vi "Actor Core.vi"(8 "error in":errorcluster, 11 "Launch IMAQ Display in":refnum<class "Launch IMAQ Display.lvclass">) -> (0 "error out":errorcluster, 3 "Actor out":refnum<class "Actor.lvclass">)   [LabVIEW 2014, in "Launch IMAQ Display.lvlib" / "Launch IMAQ Display.lvclass"]
doc: "(<B>Filename</B>: Actor Framework.lvlib:Actor.lvclass:Actor Core.vi)\n\nReceives messages to the actor, reacts to them, and initiates any error handling that may shut the actor down.\n\nDescendant classes may override this VI to append parallel tasks for the actor to complete while it handles messages. Overrides use the Call Parent Method node."
uses:
  Launch IMAQ Display.lvclass
  <vilib>/ActorFramework/Actor/Actor.lvclass
  HIJ IMAQdx Display/AF IMAQ Display/HIJ IMAQdx Display.lvclass
  Analyze Classes/Analyze Diviation/Analyze BeamDeviation.lvclass
  Results and Overlays/Results Beam Deviation/Analyze Results Beam Deviation.lvclass
  Analyze Classes/Analyze Distanz/Analyze Distanz.lvclass
  Results and Overlays/Results Distance/Analyze Results Distanz.lvclass
  IMAQdx Actor/IMAQdx Actor/IMAQdx Actor.lvclass
  Analyze Classes/Analyze Fluence/Analyze Fluence.lvclass
  Results and Overlays/Results Fluence/Analyze Results Fluence.lvclass
  Results and Overlays/Results Base/Analyze Results Base.lvclass/Analyze Results Base.ctl
  Results and Overlays/Results Fluence/Analyze Results Fluence.lvclass/Analyze Results Fluence.ctl
  HIJ Vision Display/HIJ Vision Display/HIJ Vision Display.lvclass/HIJ Vision Display.ctl
  Applications/HIJ Vision Application/HIJ Vision Application/HIJ Vision Application.lvclass/HIJ Vision Application.ctl
  Applications/HIJ Vision Camera App/HIJ Vision Camera App/HIJ Vision Camera App.lvclass/HIJ Vision Camera App.ctl
  <vilib>/ActorFramework/Actor/Actor.lvclass/Actor.ctl
  <vilib>/ActorFramework/Message Enqueuer/Message Enqueuer.lvclass/Message Enqueuer.ctl
  Applications/HIJ Vision Camera App/HIJ Vision Camera App Messages/Menu Selection Msg/Menu Selection Msg.lvclass/Menu Selection Msg.ctl
  Results and Overlays/Results Base/Write Overlay_.vi
  Results and Overlays/Results Base/Write Overlay colors.vi
  Results and Overlays/Results Fluence/Write UI Ref Max F.vi
  HIJ Vision Display/HIJ Vision Display/Write Save Report_.vi
  Applications/HIJ Vision Application/HIJ Vision Application/Write SubPnl for Display.vi
  Applications/HIJ Vision Camera App/HIJ Vision Camera App/Write Child Menu.vi
  Applications/HIJ Vision Application/HIJ Vision Application/Write HIJ Vision Display.vi
  Applications/HIJ Vision Application/HIJ Vision Application/Write Analyze Objs.vi
  Applications/HIJ Vision Camera App/HIJ Vision Camera App/Write Camera Actor.vi
  Applications/HIJ Vision Camera App/HIJ Vision Camera App/Write SubPnl for Settings.vi
  <vilib>/ActorFramework/Message Enqueuer/Init from Existing Queue.vi
  <vilib>/ActorFramework/Message Enqueuer/Enqueue.vi
  <vilib>/ActorFramework/Message Priority Queue/Priority Enqueue.vi
  <vilib>/ActorFramework/Message Enqueuer/Message Enqueuer.lvclass
  Applications/HIJ Vision Camera App/HIJ Vision Camera App Messages/Menu Selection Msg/Menu Selection Msg.lvclass
  <vilib>/ActorFramework/Stop Msg/Stop Msg.lvclass
  Applications/HIJ Vision Camera App/HIJ Vision Camera App/HIJ Vision Camera App.lvclass
panel:
  out "Max Fluence":dbl[unit]
  in  "Stop Button":bool
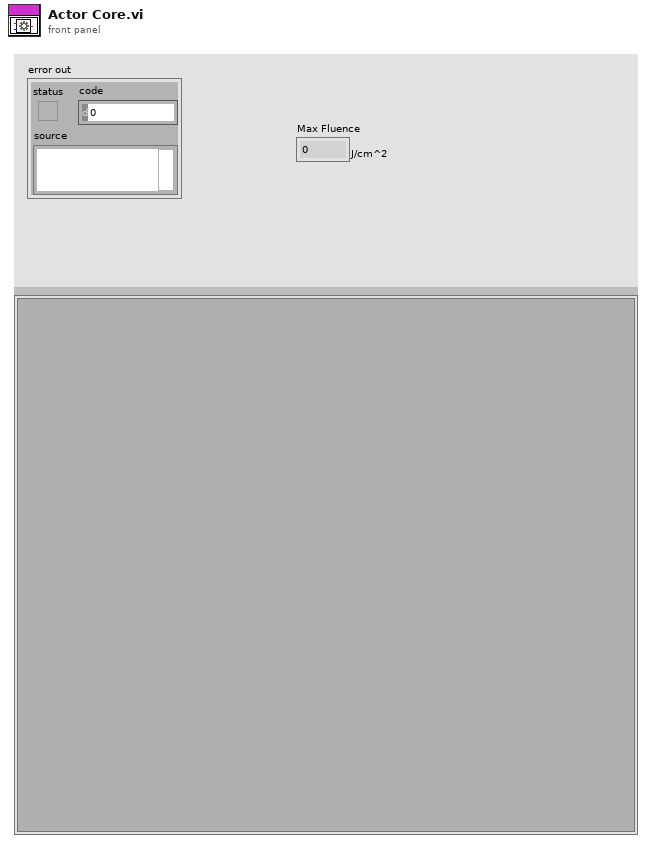
[diagram p1: front panel]
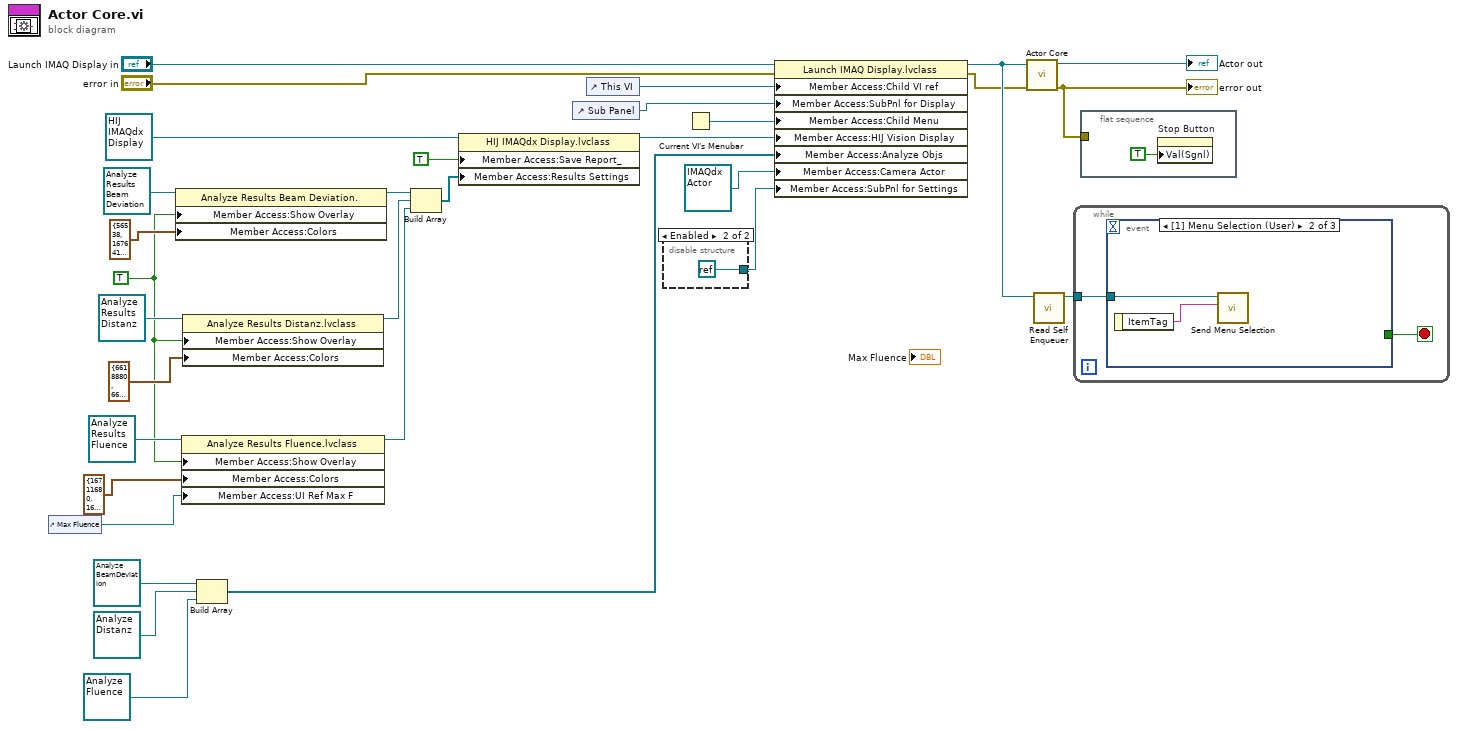
[diagram p0: block diagram]
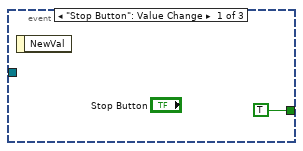
[diagram p3: hidden frame]
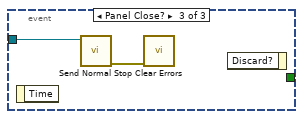
[diagram p4: hidden frame]
diagram:
  w3 = TRUE ("bOverlay")
  n1 = control-ref of="Max Fluence"() -> (w1:refnum<vi>)
  n2 = property class="Analyze Results Beam Deviation."(reference=refnum<class "Analyze Results Beam Deviation.lvclass"> refnum ("Analyze Results Beam Deviation.lvclass"), "Member Access:Show Overlay"=w3, "Member Access:Colors"=cluster{"Border":u32, "Text":u32} {"Border"=56538, "Text"=16764160} ("Colors")) -> (reference out=w23:refnum<class "Analyze Results Beam Deviation.lvclass">)  [unwired: 1 in, 1 out]
  n3 = property class="Analyze Results Fluence.lvclass"(reference=refnum<class "Analyze Results Fluence.lvclass"> refnum ("Analyze Results Fluence.lvclass"), "Member Access:Show Overlay"=w3, "Member Access:Colors"=cluster{"Border":u32, "Text":u32} {"Border"=16711680, "Text"=16448250} ("Colors"), "Member Access:UI Ref Max F"=w1) -> (reference out=w4:refnum<class "Analyze Results Fluence.lvclass">)  [unwired: 1 in, 1 out]
  n4 = property class="Analyze Results Distanz.lvclass"(reference=refnum<class "Analyze Results Distanz.lvclass"> refnum ("Analyze Results Distanz.lvclass"), "Member Access:Show Overlay"=w3, "Member Access:Colors"=cluster{"Border":u32, "Text":u32} {"Border"=6618880, "Text"=6618880} ("Colors")) -> (reference out=w18:refnum<class "Analyze Results Distanz.lvclass">)  [unwired: 1 in, 1 out]
  n5 = Build Array(refnum<class "Analyze BeamDeviation.lvclass"> refnum ("Analyze.lvlib:Analyze BeamDeviation.lvclass"), refnum<class "Analyze Distanz.lvclass"> refnum ("Analyze.lvlib:Analyze Distanz.lvclass"), refnum<class "Analyze Fluence.lvclass"> refnum ("Analyze.lvlib:Analyze Fluence.lvclass")) -> (w12:refnum<class "Analyze BaseClass.lvclass">[])
  n6 = Build Array(w23, w18, w4) -> (w22:refnum<class "Analyze Results Base.lvclass">[])
  n7 = property class="HIJ IMAQdx Display.lvclass"(reference=refnum<class "HIJ IMAQdx Display.lvclass"> refnum ("IMAQ Display.lvlib:IMAQ Display.lvclass"), "Member Access:Save Report_"=TRUE ("Save Report_"), "Member Access:Results Settings"=w22) -> (reference out=w8:refnum<class "HIJ IMAQdx Display.lvclass">)  [unwired: 1 in, 1 out]
  n8 = control-ref of="Sub Panel"() -> (w11:refnum<vi>)
  n9 = control-ref of="This VI"() -> (w15:refnum<vi>)
  n10 = disable-structure shown="Enabled" {
    disable-tunnel: [_ refnum<k0> refnum] -> w9
    frame Disabled {
    }
    frame Enabled {
    }
  }
  n11 = Current VI's Menubar() -> (w7:refnum<k9>)
  n12 = property class="Launch IMAQ Display.lvclass"(reference="Launch IMAQ Display in", error in="error in", "Member Access:Child VI ref"=w15, "Member Access:SubPnl for Display"=w11, "Member Access:Child Menu"=w7, "Member Access:HIJ Vision Display"=w8, "Member Access:Analyze Objs"=w12, "Member Access:Camera Actor"=refnum<class "IMAQdx Actor.lvclass"> refnum ("IMAQdx Actor.lvlib:IMAQdx Actor.lvclass"), "Member Access:SubPnl for Settings"=w9) -> (reference out=w16:refnum<class "Launch IMAQ Display.lvclass">, error out=w13:errorcluster)
  n13 = call-parent "Actor Core.vi"("error in"=w13, "Launch IMAQ Display in"=w16) -> ("error out"=w29:errorcluster, "Actor out"=→"Actor out":refnum<class "Actor.lvclass">)  [unwired: 8 in]
  "error out" <- w29
  n14 = call <vilib>:"Read Self Enqueuer.vi"("Actor"=w16) -> ("Self Enqueuer"=w28:refnum<class "Message Enqueuer.lvclass">)  [unwired: 10 in]
  n15 = while {
    tunnel: w28 -> [w33]
    stop <- w34 stop-if-true
    n16 = event shown="[1] Menu Selection (User)" {
      selector: _ -> [_ _ _]
      dyn-events: _ -> [_ _ _]
      timeout: _ -> [_ _ _]
      tunnel: [TRUE _ _] -> w34
      tunnel: w33 -> [_ w36 w39]
      event "Stop Button": Value Change {
        n17 = event-data() -> ()  [unwired: 1 in, 1 out]
      }
      event Menu Selection (User) {
        n18 = event-data() -> ("ItemTag"=w37:string)  [unwired: 1 in]
        n19 = call "Send Menu Selection.vi"("MenuTag"=w37, "Message Enqueuer"=w36) -> ()  [unwired: 8 in, 2 out]
      }
      event Panel Close? {
        n20 = event-data() -> ()  [unwired: 1 in, 1 out]
        n21 = call <vilib>:"Send Normal Stop.vi"("Message Enqueuer"=w39) -> ("error out"=w38:errorcluster)  [unwired: 10 in]
        n22 = call <vilib>:"Clear Errors.vi"("error in (no error)"=w38) -> ()  [unwired: 5 in, 2 out]
        n23 = event-data() -> ()  [unwired: 2 in, 1 out]
      }
    }
  }
  n24 = flat-sequence {
    tunnel: w29 -> [_]
    frame #0 {
      n25 = property on="Stop Button" class="Bool (strict)"("Val(Sgnl)"=TRUE) -> ()  [unwired: 2 in, 2 out]
    }
  }
